vi "Main.vi"() -> ()   [LabVIEW 2018, in "6509.lvlib"]
doc: "This template is based off of the Queued Message Handler design pattern and the Queued Message Handler project template that ships with LabVIEW.\n\nThe main difference is that the queue is private to this module and communication between modules is performed via Broadcast and Request events.\n\nRequest events are wrapped in public API methods and are handled in the Event Handling Loop (EHL) of this VI. Any module can register for Broadcast events sent by this module. The EHL generates messages based on user interface actions.\n\nThe Message Handling Loop (MHL) processes messages generated by the EHL, or by other messages. The messages are string values, so new messages can be added easily to the Message Cases case structure in the MHL. Each message cluster can also provide an optional value for Message Data, which is a variant that can be converted to whatever message-specific data is required.\n_____\nBased on Delacor QMH Project Template 4.2.1.64."
uses:
  6509.lvlib
  Module Data--cluster.ctl
  <vilib>/Delacor/Delacor QMH/Libraries/Message Queue_class/Delacor_lib_QMH_Message Queue.lvclass
  <vilib>/Delacor/Delacor QMH/Libraries/Message Queue_class/Delacor_lib_QMH_Enqueue Message (Single).vi
  <vilib>/ErrorRing/Error Ring.xnode
  <vilib>/Utility/error.llb/Error Cluster From Error Code.vi
  <vilib>/Delacor/Delacor QMH/Libraries/Module Admin_class/Delacor_lib_QMH_Module Admin.lvclass
  Stop Argument--cluster.ctl
  <vilib>/Utility/miscctls.llb/LVPointTypeDef.ctl
  Start Edge Detection (Reply Payload)--cluster.ctl
  Start Edge Detection Argument--cluster.ctl
  Stop Edge Detection Argument--cluster.ctl
panel:
  in  "lines in":tag="Dev1/port8/line6:7"
  in  "file in":path=path "C:/my_work/labview_work/dqmh/d_6509/Counter/spill_id.txt"
  out "error out":errorcluster
  in  "Module Admin":refnum<class "Delacor_lib_QMH_Module Admin.lvclass">
  out "Status":string
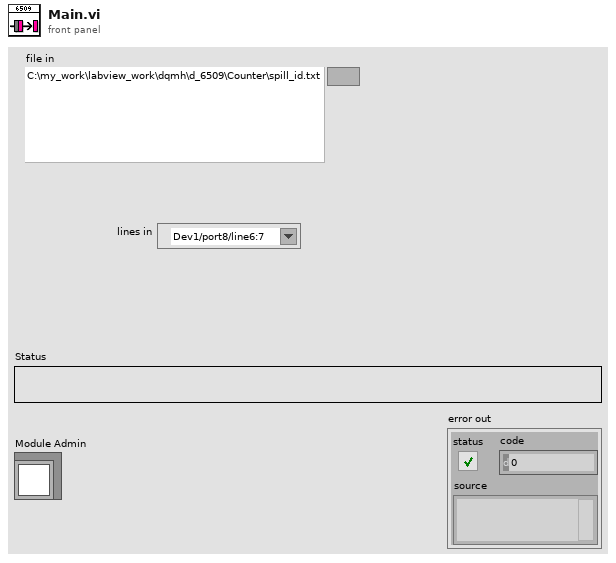
[diagram p1: front panel]
types:
  T1 = typedef "6509.lvlib/Request Events--cluster.ctl" = cluster{"Stop Module":refnum<user-event>, "Show Panel":refnum<user-event>, "Hide Panel":refnum<user-event>, "Get Module Execution Status":refnum<user-event>, "Show Diagram":refnum<user-event>, "Wakeup Helper Loop":refnum<user-event>, "Start Edge Detection":refnum<user-event>, "Stop Edge Detection":refnum<user-event>, "Pass Settings 4Helper":refnum<user-event>}
  T2 = cluster{"Event Registration Refnum":refnum<event-registration>, "Event Registration Refnum":refnum<event-registration>}
  T3 = enum32{"invalid lock state", "Not Locked", "Locked (No Password)", "Password-protected"}
  T4 = typedef "6509.lvlib/Stop Argument--cluster.ctl" = cluster{"Origin":string, "Exit via Stop Module Req?":bool, "Wait for Module to stop?":bool}
  T5 = typedef "6509.lvlib/Start Edge Detection Argument--cluster.ctl" = cluster{"arg_spare":bool, "Wait Notifier":refnum<notifier>, "wait for reply":bool}
  T6 = typedef "6509.lvlib/Stop Edge Detection Argument--cluster.ctl" = cluster{"arg_spare":bool}
  T7 = typedef "LVPointTypeDef.ctl" = cluster{"Horizontal":i16, "Vertical":i16}
  T8 = enum32{"Invalid", "Standard", "Closed", "Hidden", "Minimized", "Maximized"}
  T9 = typedef "6509.lvlib/Start Edge Detection (Reply Payload)--cluster.ctl" = cluster{"device_task":refnum<k21>, "Start Edge Detection_error":errorcluster}
  T10 = typedef "6509.lvlib/Module Data--cluster.ctl" = cluster{"Status":string, "task":refnum<k21>, "file in":path, "get_sid":u32}
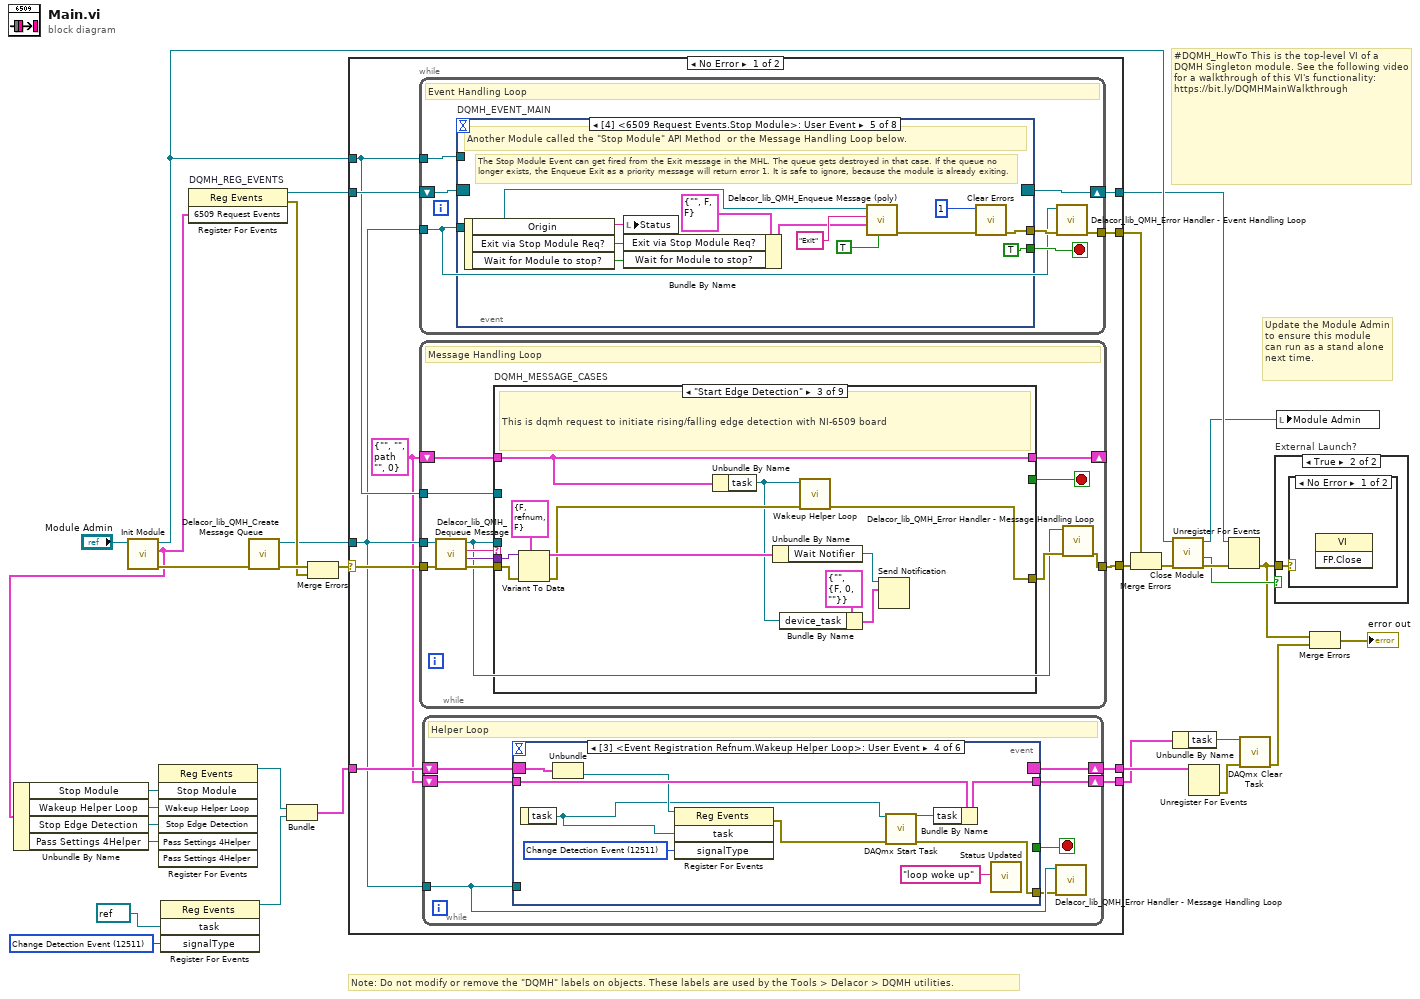
[diagram p0: block diagram]
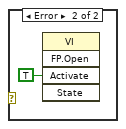
[diagram p3: hidden frame]
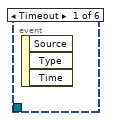
[diagram p4: hidden frame]
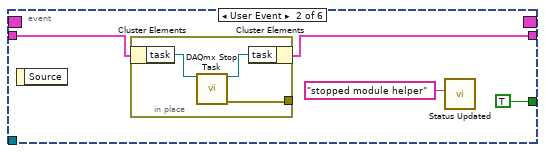
[diagram p5: hidden frame]
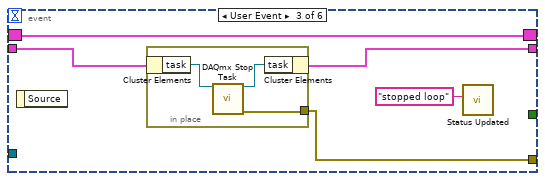
[diagram p6: hidden frame]
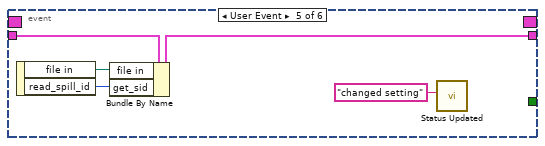
[diagram p7: hidden frame]
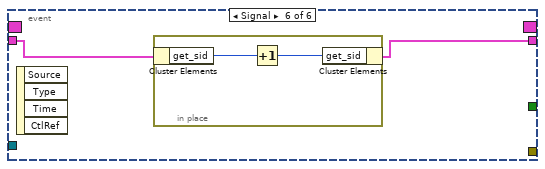
[diagram p8: hidden frame]
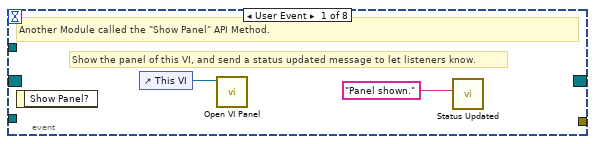
[diagram p9: hidden frame]
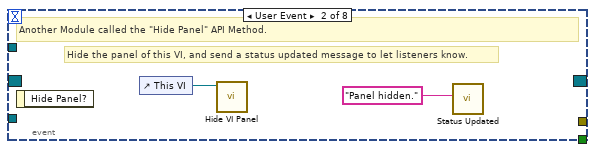
[diagram p10: hidden frame]
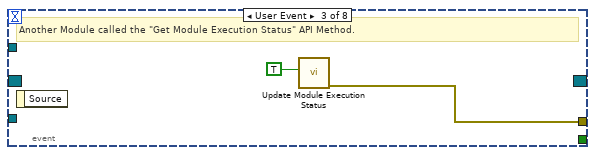
[diagram p11: hidden frame]
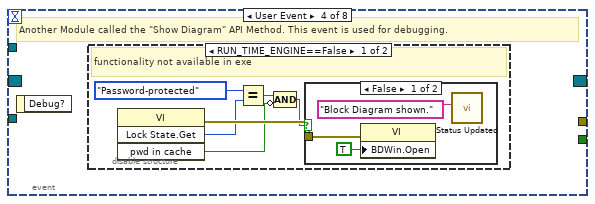
[diagram p12: hidden frame]
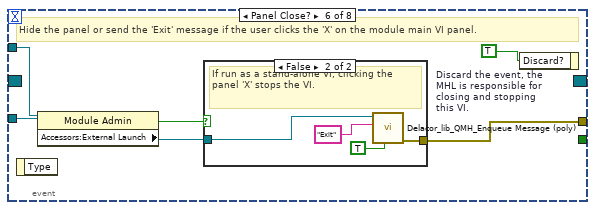
[diagram p15: hidden frame]
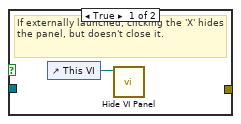
[diagram p16: hidden frame]
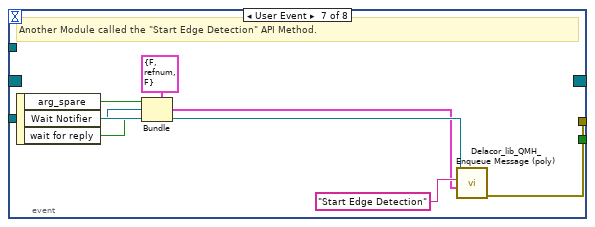
[diagram p17: hidden frame]
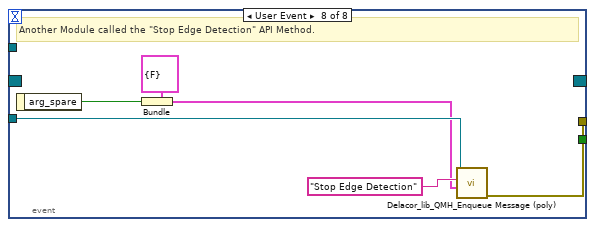
[diagram p18: hidden frame]
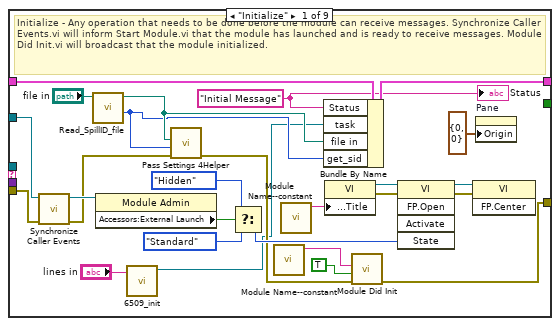
[diagram p19: hidden frame]
diagram:
  w4 = 12511 items=["Sample Complete Event"=12530, "Counter Output Event"=12494, "Change Detection Event"=12511, "Sample Clock"=12487] ("signalType")
  # "#DQMH_HowTo This is the top-level VI of a DQMH Singleton module. See the following video for a walkthrough of this VI's functionality: https://bit.ly/DQMHMainWalkthrough"
  # "Note: Do not modify or remove the \"DQMH\" labels on objects. These labels are used by the Tools > Delacor > DQMH utilities."
  # "Update the Module Admin to ensure this module can run as a stand alone next time."
  n1 = call "Init Module.vi"("Singleton Module Admin in"="Module Admin") -> ("error out"=w31:errorcluster, "6509 Request Events"=w17:T1, "Singleton Module Admin out"=w24:refnum<class "Delacor_lib_QMH_Module Admin.lvclass">)  [unwired: 8 in]
  n2 = Unbundle By Name(w17) -> ("Stop Module"=w16:refnum<user-event>, "Wakeup Helper Loop"=w12:refnum<user-event>, "Stop Edge Detection"=w11:refnum<user-event>, "Pass Settings 4Helper"=w10:refnum<user-event>)
  n3 = register-events(w16, w12, w11, w10) -> (reference out=w3:refnum<event-registration>)  [unwired: 3 in, 1 out]
  n4 = register-events(refnum<k21> refnum ("task"), w4) -> (reference out=w2:refnum<event-registration>)  [unwired: 2 in, 1 out]
  n5 = register-events "DQMH_REG_EVENTS"(w17) -> (reference out=w22:refnum<event-registration>, error out=w25:errorcluster)  [unwired: 2 in]
  n6 = call <vilib>:"Delacor_lib_QMH_Create Message Queue.vi"("error in (no error)"=w31) -> ("error out"=w27:errorcluster, "Message Queue"=w21:refnum<class "Delacor_lib_QMH_Message Queue.lvclass">)  [unwired: 9 in]
  n7 = Bundle("Event Registration Refnum"=w3, "Event Registration Refnum"=w2) -> (w1:T2)  [unwired: 1 in]
  n8 = Merge Errors(w27, w25) -> (w26:errorcluster)
  n9 = case shown="No Error" w26 {
    selector: w26 -> [w41 w259]
    tunnel: [w43 w259] -> w32
    tunnel: [w40 w256] -> w23
    tunnel: w22 -> [w39 w256]
    tunnel: w21 -> [w36 _]
    tunnel: [w42 _] -> w29
    tunnel: w24 -> [w38 w252]
    tunnel: w1 -> [w37 w251]
    tunnel: [w35 w251] -> w15
    tunnel: [w33 T10 {"Status"="", "task"="", "file in"=path "", "get_sid"=0} ("Data Cluster")] -> w9
    frame No Error {
      w34 = T10 {"Status"="", "task"="", "file in"=path "", "get_sid"=0} ("Data Cluster")
      n10 = while {
        tunnel: w36 -> [w85]
        shift-right: [w88] -> w40
        shift-left: w39 -> [w89]
        tunnel: [w90] -> w42
        tunnel: w38 -> [w86]
        stop <- w87 stop-if-true
        # "Event Handling Loop"
        n11 = event "DQMH_EVENT_MAIN" shown="[4] <6509 Request Events.Stop Module>: User Event" {
          selector: w89 -> [_ _ _ _ _ _ _ _]
          dyn-events: [_ _ _ _ _ _ _ _] -> w88
          timeout: _ -> [_ _ _ _ _ _ _ _]
          tunnel: [_ _ _ _ TRUE ("Discard?") _ _ _] -> w87
          tunnel: w85 -> [_ _ _ _ w114 w121 w136 w142]
          tunnel: [_ _ w97 _ w117 w123 w129 w137] -> w91
          tunnel: w86 -> [_ _ _ _ _ w120 _ _]
          event User Event {
            # "Show the panel of this VI, and send a status updated message to let listeners know."
            # "Another Module called the \"Show Panel\" API Method."
            n12 = event-data() -> ()  [unwired: 1 in, 1 out]
            n13 = control-ref of="This VI"() -> (w93:refnum<vi>)
            n14 = call "Open VI Panel.vi"("VI"=w93) -> ()  [unwired: 10 in, 1 out]
            n15 = call "Status Updated.vi"("Status"="Panel shown." ("format string")) -> ()  [unwired: 10 in, 1 out]
          }
          event User Event {
            # "Hide the panel of this VI, and send a status updated message to let listeners know."
            # "Another Module called the \"Hide Panel\" API Method."
            n16 = event-data() -> ()  [unwired: 1 in, 1 out]
            n17 = control-ref of="This VI"() -> (w95:refnum<vi>)
            n18 = call "Hide VI Panel.vi"("VI"=w95) -> ()  [unwired: 10 in, 1 out]
            n19 = call "Status Updated.vi"("Status"="Panel hidden." ("format string")) -> ()  [unwired: 10 in, 1 out]
          }
          event User Event {
            # "Another Module called the \"Get Module Execution Status\" API Method."
            n20 = event-data() -> ()  [unwired: 1 in, 1 out]
            n21 = call "Update Module Execution Status.vi"("Running?"=TRUE) -> ("error out"=w97:errorcluster)  [unwired: 10 in]
          }
          event User Event {
            # "Another Module called the \"Show Diagram\" API Method. This event is used for debugging."
            n22 = event-data() -> ()  [unwired: 1 in, 1 out]
            n23 = disable-structure shown="RUN_TIME_ENGINE==False" {
              frame condition #0 (active) {
                # "functionality not available in exe"
                n24 = invoke class="VI" method="Lock State.Get"() -> (error out=w103:errorcluster, "Get Lock State"=w102:T3, "pwd in cache"=w99:bool)  [unwired: 4 in, 1 out]
                n25 = Equal?(x=T3."Password-protected", y=w102) -> (x = y?=w100:bool)
                n26 = Compound Arithmetic op=AND(w100, invert w99) -> (w98:bool)
                n27 = case shown="False" w98 {
                  tunnel: w103 -> [w106 _]
                  frame False {
                    n28 = property class="VI"(error in=w106, "BDWin.Open"=TRUE ("Block Diagram Window:Open")) -> ()  [unwired: 1 in, 2 out]
                    n29 = call "Status Updated.vi"("Status"="Block Diagram shown." ("format string")) -> ()  [unwired: 10 in, 1 out]
                  }
                  frame True {
                    # "Password-protected VI, and the password is not in the cache. Do not show the diagram."
                  }
                }
              }
              frame condition #1 {
              }
            }
          }
          event User Event {
            # "The Stop Module Event can get fired from the Exit message in the MHL. The queue gets destroyed in that case. If the queue no longer exists, the Enqueue Exit as a priority message will return error 1. It is safe to ignore, because the module is already exiting."
            # "Another Module called the \"Stop Module\" API Method  or the Message Handling Loop below."
            n30 = event-data() -> ("Origin"=w113:string, "Exit via Stop Module Req?"=w109:bool, "Wait for Module to stop?"=w108:bool)  [unwired: 1 in]
            n31 = local write "Status"(w113) -> ()
            n32 = Bundle By Name(cluster=T4 {"Origin"="", "Exit via Stop Module Req?"=FALSE, "Wait for Module to stop?"=FALSE} ("Stop Argument"), "Exit via Stop Module Req?"=w109, "Wait for Module to stop?"=w108) -> (w107:T4)
            n33 = call-poly <vilib>:"Delacor_lib_QMH_Enqueue Message (poly).vi"("Priority Message? (F)"=TRUE, "Message Data"=w107, "Message"="Exit", "Message Queue in"=w114) -> ("error out"=w118:errorcluster)  [unwired: 6 in, 1 out]
            n34 = call <vilib>:"Clear Errors.vi"("error in (no error)"=w118, "specific error code to clear (0: all)"=1) -> ("error out"=w117:errorcluster)  [unwired: 4 in, 1 out]
          }
          event Panel Close? {
            w122 = TRUE  # Discard the event, the MHL is responsible for closing and stopping this VI.
            # "Hide the panel or send the 'Exit' message if the user clicks the 'X' on the module main VI panel."
            n35 = event-data() -> ()  [unwired: 1 in, 1 out]
            n36 = property class="Module Admin"(reference=w120) -> ("Accessors:External Launch"=w119:bool)  [unwired: 1 in, 2 out]
            n37 = case shown="False" w119 {
              tunnel: w121 -> [_ w127]
              tunnel: [_ w128] -> w123
              frame True {
                # "If externally launched, clicking the 'X' hides the panel, but doesn't close it."
                n38 = control-ref of="This VI"() -> (w124:refnum<vi>)
                n39 = call "Hide VI Panel.vi"("VI"=w124) -> ()  [unwired: 10 in, 1 out]
              }
              frame False {
                # "If run as a stand-alone VI, clicking the panel 'X' stops the VI."
                n40 = call-poly <vilib>:"Delacor_lib_QMH_Enqueue Message (poly).vi"("Priority Message? (F)"=TRUE, "Message"="Exit", "Message Queue in"=w127) -> ("error out"=w128:errorcluster)  [unwired: 7 in, 1 out]
              }
            }
            n41 = event-data("Discard?"=w122) -> ()  [unwired: 1 in, 1 out]
          }
          event User Event {
            # "Another Module called the \"Start Edge Detection\" API Method."
            n42 = event-data() -> ("arg_spare"=w132:bool, "Wait Notifier"=w131:refnum<notifier>, "wait for reply"=w130:bool)  [unwired: 1 in]
            n43 = Bundle(cluster=T5 {"arg_spare"=FALSE, "Wait Notifier"=refnum, "wait for reply"=FALSE} ("Start Edge Detection Argument"), "arg_spare"=w132, "Wait Notifier"=w131, "wait for reply"=w130) -> (w133:T5)
            n44 = call-poly <vilib>:"Delacor_lib_QMH_Enqueue Message (poly).vi"("Message Data"=w133, "Message"="Start Edge Detection", "Message Queue in"=w136) -> ("error out"=w129:errorcluster)  [unwired: 7 in, 1 out]
          }
          event User Event {
            # "Another Module called the \"Stop Edge Detection\" API Method."
            n45 = event-data() -> ("arg_spare"=w138:bool)  [unwired: 1 in]
            n46 = Bundle(cluster=T6 {"arg_spare"=FALSE} ("Stop Edge Detection Argument"), "arg_spare"=w138) -> (w139:T6)
            n47 = call-poly <vilib>:"Delacor_lib_QMH_Enqueue Message (poly).vi"("Message Data"=w139, "Message"="Stop Edge Detection", "Message Queue in"=w142) -> ("error out"=w137:errorcluster)  [unwired: 7 in, 1 out]
          }
        }
        n48 = call-dynamic "Delacor_lib_QMH_Error Handler - Event Handling Loop.vi"("error in (no error)"=w91, "Message Queue in"=w85) -> ("dup error in"=w90:errorcluster)  [unwired: 8 in, 1 out]
      }
      n49 = while {
        tunnel: w36 -> [w145]
        shift-right: [w149] -> _
        shift-left: w34 -> [w150]
        tunnel: w41 -> [w153]
        tunnel: [w151] -> w43
        tunnel: w38 -> [w143]
        stop <- w148 stop-if-true
        # "Message Handling Loop"
        n50 = call-dynamic "Delacor_lib_QMH_Dequeue Message.vi"("error in (no error)"=w153, "Message Queue in"=w145) -> ("error out"=w152:errorcluster, "Message Data"=w146:variant, "Message"=w147:string, "Message Queue out"=w144:refnum<class "Delacor_lib_QMH_Message Queue.lvclass">)  [unwired: 6 in]
        n51 = case "DQMH_MESSAGE_CASES" shown="\"Start Edge Detection\"" w147 {
          selector: w147 -> [_ _ _ _ _ _ _ _ w237]
          tunnel: w144 -> [_ _ _ _ _ _ w207 w229 _]
          tunnel: w152 -> [w178 w182 w193 w199 w202 w204 w214 w235 w239]
          tunnel: [w177 w182 w186 w194 w201 w204 w210 w232 w240] -> w154
          tunnel: w150 -> [w168 w181 w185 w195 w200 w203 w209 w228 w238]
          tunnel: [w167 w181 w185 w195 w200 w203 w209 w228 w238] -> w149
          tunnel: [_ _ _ _ _ _ _ w227 _] -> w148
          tunnel: w146 -> [_ _ w192 w198 _ _ w208 w226 _]
          tunnel: w143 -> [w169 _ _ _ _ _ w206 w221 _]
          frame "Initialize" {
            w162 = "Initial Message" ("Initial Message")
            # "Initialize - Any operation that needs to be done before the module can receive messages. Synchronize Caller Events.vi will inform Start Module.vi that the module has launched and is ready to receive messages. Module Did Init.vi will broadcast that the module initialized."
            n52 = call "Synchronize Caller Events.vi"("error in (no error)"=w178, "Singleton Module Admin in"=w169) -> ("error out"=w160:errorcluster, "Singleton Module Admin out"=w164:refnum<class "Delacor_lib_QMH_Module Admin.lvclass">)  [unwired: 8 in]
            n53 = call "Read_SpillID_file.vi"("file in"="file in") -> ("get_sid"=w157:u32, "file out"=w158:path)  [unwired: 7 in, 2 out]
            n54 = property class="Module Admin"(reference=w164) -> ("Accessors:External Launch"=w173:bool)  [unwired: 1 in, 2 out]
            n55 = call "6509_init.vi"("lines in"="lines in") -> ("task out"=w155:refnum<k21>)  [unwired: 8 in, 2 out]
            n56 = call "Pass Settings 4Helper.vi"("error in (no error)"=w160, "get_sid"=w157, "file in"=w158) -> ("error out"=w159:errorcluster)  [unwired: 8 in]
            n57 = Select(t=T8."Hidden" ("State"), s=w173, f=T8."Standard" ("State")) -> (s? t:f=w170:T8)
            n58 = call "Module Name--constant.vi"() -> ("Module Name"=w165:string)  [unwired: 11 in]
            n59 = call "Module Name--constant.vi"() -> ("Module Name"=w176:string)  [unwired: 11 in]
            n60 = Bundle By Name(cluster=w168, "Status"=w162, "task"=w155, "file in"=w158, "get_sid"=w157) -> (w167:T10)
            n61 = property class="VI"("Front Panel.Title"=w176) -> (reference out=w175:refnum<vi>, error out=w180:errorcluster)  [unwired: 2 in]
            n62 = call "Module Did Init.vi"("error in (no error)"=w159, "Initialized?"=TRUE, "Origin"=w165) -> ("error out"=w177:errorcluster)  [unwired: 8 in]
            n63 = invoke class="VI" method="FP.Open"(reference=w175, error in=w180, "State"=w170) -> (reference out=w174:refnum<vi>, error out=w179:errorcluster)  [unwired: 2 in, 3 out]
            n64 = invoke class="VI" method="FP.Center"(reference=w174, error in=w179) -> ()  [unwired: 1 in, 3 out]
            n65 = property on="Pane" class="Pane"("Origin"=T7 {"Horizontal"=0, "Vertical"=0}) -> ()  [unwired: 2 in, 2 out]
            "Status" <- w162
          }
          frame "--- Module Specific ---" {
            # "Separator -- The following cases handle messages specific to this Module."
          }
          frame "Start Edge Detection" {
            # "This is dqmh request to initiate rising/falling edge detection with NI-6509 board"
            n66 = Variant To Data(error in=w193, type=T5 {"arg_spare"=FALSE, "Wait Notifier"=refnum, "wait for reply"=FALSE} ("Start Edge Detection Argument"), Variant=w192) -> (data=w190:T5, error out=w184:errorcluster)
            n67 = Unbundle By Name(w185) -> ("task"=w183:refnum<k21>)
            n68 = Unbundle By Name(w190) -> ("Wait Notifier"=w189:refnum<notifier>)
            n69 = Bundle By Name(cluster=T9 {"device_task"="", "Start Edge Detection_error"={"status"=FALSE, "code"=0, "source"=""}} ("Start Edge Detection (Reply Payload)"), "device_task"=w183) -> (w188:T9)
            n70 = call "Wakeup Helper Loop.vi"("error in (no error)"=w184, "task"=w183) -> ("error out"=w186:errorcluster)  [unwired: 9 in]
            n71 = Send Notification(notification=w188, notifier=w189) -> ()  [unwired: 1 in, 2 out]
          }
          frame "Stop Edge Detection" {
            # "This is dqmh request to stop detection of the rising/falling edges with NI-6509 board"
            n72 = Variant To Data(error in=w199, type=T6 {"arg_spare"=FALSE} ("Stop Edge Detection Argument"), Variant=w198) -> (error out=w194:errorcluster)  [unwired: 1 out]
            n73 = Unbundle By Name(w195) -> ()  [unwired: 1 out]
            n74 = call "Status Updated.vi"("Status"="stopped daq") -> ()  [unwired: 10 in, 1 out]
          }
          frame "---Copy This Frame---" {
            # "Duplicate this frame when creating new messages.  Change this comment in the duplicated frame to describe this message."
            n75 = Merge Errors(w202) -> (w201:errorcluster)
          }
          frame "--- Exit and Error Handling---" {
            # "Separator - The following cases handle errors and exit messages."
          }
          frame "Error" {
            # "Error - Check the error message data and respond accordingly. This message is sent by the \"Error Handler\" VIs at the end of each loop in this application."
            n76 = property class="Module Admin"(reference=w206) -> ("Accessors:External Launch"=w205:bool)  [unwired: 1 in, 2 out]
            n77 = Variant To Data(error in=w214, type=errorcluster {"status"=FALSE, "code"=0, "source"=""} ("error constant"), Variant=w208) -> (data=w215:errorcluster, error out=w212:errorcluster)
            n78 = call "Error Reported.vi"("Error"=w215) -> ()  [unwired: 10 in, 1 out]
            n79 = case shown="False" w205 {
              tunnel: [w220 _] -> w211
              tunnel: w207 -> [w218 _]
              tunnel: w215 -> [w219 _]
              frame False {
                # "If the module is running standalone, then pop up an error dialog and call the \"Exit\" message."
                n80 = call <vilib>:"Simple Error Handler.vi"("error in (no error)"=w219) -> ()  [unwired: 4 in, 5 out]
                n81 = call-poly <vilib>:"Delacor_lib_QMH_Enqueue Message (poly).vi"("Priority Message? (F)"=TRUE, "Message"="Exit", "Message Queue in"=w218) -> ("error out"=w220:errorcluster)  [unwired: 7 in, 1 out]
              }
              frame True {
                # "If the module was launched externally, calling the Error Reported broadcast VI is the only action performed by the \"Error\" message. The module's caller can then process the error appropriately."
              }
            }
            n82 = Merge Errors(w212, w211) -> (w210:errorcluster)
            n83 = local write "error out"(w210) -> ()
          }
          frame "Exit" {
            w225 = 91  # 91: not all Exit messages will have an argument
            w227 = TRUE  # Stop the VI
            # "Release the message queue reference"
            # "Exit - Exit the application."
            n84 = Variant To Data(error in=w235, type=T4 {"Origin"="", "Exit via Stop Module Req?"=FALSE, "Wait for Module to stop?"=FALSE} ("Stop Argument"), Variant=w226) -> (data=w223:T4, error out=w231:errorcluster)
            n85 = call <vilib>:"Clear Errors.vi"("error in (no error)"=w231, "specific error code to clear (0: all)"=w225) -> ("error out"=w234:errorcluster)  [unwired: 4 in, 1 out]
            n86 = control-ref of="This VI"() -> (w222:refnum<vi>)
            n87 = call-dynamic "Delacor_lib_QMH_Release Message Queue.vi"("error in (no error)"=w234, "Message Queue"=w229) -> ("error out"=w233:errorcluster)  [unwired: 9 in]
            n88 = call "Handle Exit.vi"("Stop Argument"=w223, "Admin in"=w221, "VI reference"=w222) -> ("error out"=w230:errorcluster)  [unwired: 7 in, 1 out]
            n89 = Merge Errors(w233, w230) -> (w232:errorcluster)
          }
          frame Default {
            # "'Default' case only runs if there is a message that isn't defined in any of the other cases.  Output a programming error."
            n90 = call "Module Name--constant.vi"() -> ("Module Name"=w236:string)  [unwired: 11 in]
            n91 = xnode "Error Ring"("parameter 0"=w237, "parameter 1"=w236) -> ("error out"=w241:errorcluster)
            n92 = Merge Errors(w239, w241) -> (w240:errorcluster)
          }
        }
        n93 = call-dynamic "Delacor_lib_QMH_Error Handler - Message Handling Loop.vi"("error in (no error)"=w154, "Message Queue in"=w144) -> ("dup error in"=w151:errorcluster)  [unwired: 8 in, 1 out]
      }
      n94 = while {
        shift-right: [w47] -> w35
        shift-left: w37 -> [w50]
        tunnel: w36 -> [w49]
        shift-right: [w45] -> w33
        shift-left: w34 -> [w46]
        stop <- w48 stop-if-true
        # "Helper Loop"
        n95 = event shown="[3] <Event Registration Refnum.Wakeup Helper Loop>: User Event" {
          selector: w50 -> [_ _ w61 w71 _ _]
          dyn-events: [_ _ w61 _ _ _] -> w47
          timeout: _ -> [_ _ _ _ _ _]
          tunnel: w49 -> [_ _ _ _ _ _]
          tunnel: [_ TRUE _ _ _ _] -> w48
          tunnel: w46 -> [_ w53 w60 w73 w79 w82]
          tunnel: [_ w52 w59 w72 w76 w81] -> w45
          tunnel: [_ _ w58 w66 _ _] -> w44
          event Timeout {
            n96 = event-data() -> ()  [unwired: 1 in, 3 out]
          }
          event User Event {
            n97 = event-data() -> ()  [unwired: 1 in, 1 out]
            n98 = in-place {
              in-place-border: [w55] -> _
              n99 = in-place-cluster #1(w53) -> ("task"=w57:refnum<k21>)
              n100 = call <vilib>:"DAQmx Stop Task.vi"("task/channels in"=w57) -> ("task out"=w56:refnum<k21>, "error out"=w55:errorcluster)  [unwired: 13 in]
              n101 = in-place-cluster #1("task"=w56) -> (w52:T10)
            }
            n102 = call "Status Updated.vi"("Status"="stopped module helper") -> ()  [unwired: 10 in, 1 out]
          }
          event User Event {
            n103 = event-data() -> ()  [unwired: 1 in, 1 out]
            n104 = in-place {
              in-place-border: [w63] -> w58
              n105 = in-place-cluster #2(w60) -> ("task"=w65:refnum<k21>)
              n106 = call <vilib>:"DAQmx Stop Task.vi"("task/channels in"=w65) -> ("task out"=w64:refnum<k21>, "error out"=w63:errorcluster)  [unwired: 13 in]
              n107 = in-place-cluster #2("task"=w64) -> (w59:T10)
            }
            n108 = call "Status Updated.vi"("Status"="stopped loop") -> ()  [unwired: 10 in, 1 out]
          }
          event User Event {
            w69 = 12511 items=["Sample Complete Event"=12530, "Counter Output Event"=12494, "Change Detection Event"=12511, "Sample Clock"=12487] ("signalType")
            n109 = event-data() -> ("task"=w68:refnum<k21>)  [unwired: 1 in]
            n110 = Unbundle(w71) -> ("Event Registration Refnum"=w70:refnum<event-registration>)  [unwired: 1 out]
            n111 = register-events(reference=w70, w68, w69) -> (error out=w67:errorcluster)  [unwired: 1 in, 1 out]
            n112 = call <vilib>:"DAQmx Start Task.vi"("task/channels in"=w68, "error in"=w67) -> ("task out"=w74:refnum<k21>, "error out"=w66:errorcluster)  [unwired: 12 in]
            n113 = Bundle By Name(cluster=w73, "task"=w74) -> (w72:T10)
            n114 = call "Status Updated.vi"("Status"="loop woke up") -> ()  [unwired: 10 in, 1 out]
          }
          event User Event {
            n115 = event-data() -> ("file in"=w78:path, "read_spill_id"=w77:u32)  [unwired: 1 in]
            n116 = Bundle By Name(cluster=w79, "file in"=w78, "get_sid"=w77) -> (w76:T10)
            n117 = call "Status Updated.vi"("Status"="changed setting") -> ()  [unwired: 10 in, 1 out]
          }
          event Signal {
            n118 = event-data() -> ()  [unwired: 1 in, 4 out]
            n119 = in-place {
              n120 = in-place-cluster #3(w82) -> ("get_sid"=w84:u32)
              n121 = Increment(x=w84) -> (x+1=w83:u32)
              n122 = in-place-cluster #3("get_sid"=w83) -> (w81:T10)
            }
          }
        }
        n123 = call-dynamic "Delacor_lib_QMH_Error Handler - Message Handling Loop.vi"("error in (no error)"=w44, "Message Queue in"=w49) -> ()  [unwired: 8 in, 2 out]
      }
    }
    frame Error {
      # "Synchronize Caller Events.vi will inform Start Module.vi that the module has launched and will let the code calling Start Module.vi register for broadcasts and would permit the caller receive the broadcast that an error occurred at launch time."
      n124 = call "Synchronize Caller Events.vi"("Singleton Module Admin in"=w252) -> ("error out"=w257:errorcluster)  [unwired: 9 in, 1 out]
      n125 = call "Module Name--constant.vi"() -> ("Module Name"=w255:string)  [unwired: 11 in]
      n126 = Format Into String(format string="An error occurred during initialization. %s is no longer running.", w255) -> (resulting string=w253:string)  [unwired: 2 in, 1 out]
      n127 = Merge Errors(w259, w257) -> (w258:errorcluster)
      n128 = call "Error Reported.vi"("Additional Information"=w253, "Error"=w258) -> ()  [unwired: 9 in, 1 out]
    }
  }
  n129 = Merge Errors(w29, w32) -> (w28:errorcluster)
  n130 = call "Close Module.vi"("error in (no error)"=w28, "Module Admin in"=w24) -> ("error out"=w30:errorcluster, "External Launch"=w18:bool, "Module Admin out"=w19:refnum<class "Delacor_lib_QMH_Module Admin.lvclass">)  [unwired: 7 in]
  n131 = Unbundle By Name(w9) -> ("task"=w8:refnum<k21>)
  n132 = Unregister For Events(event registration refnum=w15) -> (error out=w7:errorcluster)  [unwired: 1 in]
  n133 = Unregister For Events(event registration refnum=w23, error in=w30) -> (error out=w14:errorcluster)
  n134 = call <vilib>:"DAQmx Clear Task.vi"("task in"=w8, "error in"=w7) -> ("error out"=w6:errorcluster)  [unwired: 13 in]
  n135 = case "External Launch?" shown="True" w18 {
    tunnel: w14 -> [_ w260]
    frame False {
    }
    frame True {
      n136 = case shown="No Error" w260 {
        frame No Error {
          n137 = invoke class="VI" method="FP.Close"() -> ()  [unwired: 3 in, 3 out]
        }
        frame Error {
          n138 = invoke class="VI" method="FP.Open"("Activate"=TRUE ("Activate?")) -> ()  [unwired: 4 in, 5 out]
        }
      }
    }
  }
  n139 = local write "Module Admin"(w19) -> ()
  n140 = Merge Errors(w14, w6) -> (→"error out":errorcluster)
